vi "BIN_File.vi"(6 "Enum":enum16{"Read", "Write"}(ring), 8 "error in":errorcluster, 10 "Data":string, 11 "Path":path) -> (0 "error out":errorcluster, 2 "data out":string)   [LabVIEW 2024, in "Launcher_DTU.lvlib"]
uses:
  Launcher_DTU.lvlib
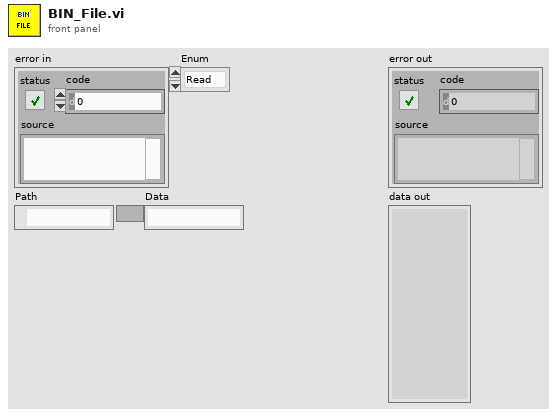
[diagram p1: front panel]
types:
  T1 = enum16{"open", "replace", "create", "open or create", "replace or create", "replace or create with confirmation"}
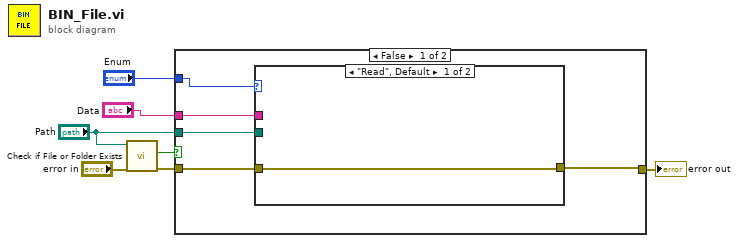
[diagram p0: block diagram]
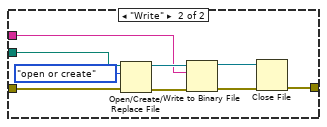
[diagram p2: hidden frame]
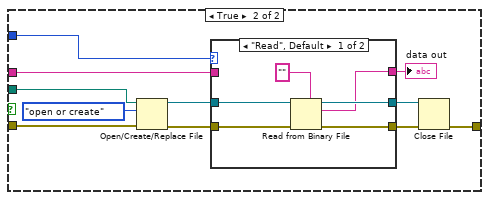
[diagram p3: hidden frame]
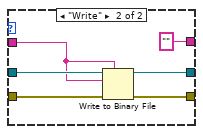
[diagram p4: hidden frame]
diagram:
  n1 = call <vilib>:"Check if File or Folder Exists.vi"("error in (no error)"="error in", "path"="Path") -> ("error out"=w6:errorcluster, "file or folder exists?"=w5:bool)  [unwired: 7 in, 1 out]
  n2 = case shown="False" w5 {
    tunnel: w6 -> [w11 w33]
    tunnel: "Path" -> [w10 w32]
    tunnel: [w8 w27] -> w3
    tunnel: "Data" -> [w9 w25]
    tunnel: "Enum" -> [w12 w24]
    frame False {
      n3 = case shown="\"Read\", Default" w12 {
        tunnel: w11 -> [w13 w22]
        tunnel: w10 -> [_ w21]
        tunnel: w9 -> [_ w17]
        tunnel: [w13 w14] -> w8
        frame "Read", Default {
        }
        frame "Write" {
          n4 = Open/Create/Replace File(file path (use dialog)=w21, error in=w22, operation (0:open)=T1."open or create") -> (refnum out=w18:refnum<file>, error out=w19:errorcluster)  [unwired: 3 in, 1 out]
          n5 = Write to Binary File(file (use dialog)=w18, data=w17, error in=w19) -> (refnum out=w16:refnum<file>, error out=w15:errorcluster)  [unwired: 3 in, 1 out]
          n6 = Close File(refnum=w16, error in=w15) -> (error out=w14:errorcluster)  [unwired: 1 out]
        }
      }
    }
    frame True {
      n7 = Open/Create/Replace File(file path (use dialog)=w32, error in=w33, operation (0:open)=T1."open or create") -> (refnum out=w28:refnum<file>, error out=w30:errorcluster)  [unwired: 3 in, 1 out]
      n8 = case shown="\"Read\", Default" w24 {
        tunnel: w30 -> [w39 w45]
        tunnel: [w38 w44] -> w29
        tunnel: w28 -> [w37 w43]
        tunnel: [w36 w42] -> w26
        tunnel: w25 -> [_ w41]
        tunnel: [w34 ""] -> w23
        frame "Read", Default {
          n9 = Read from Binary File(5:"" ("data type"), 8:w39, 11:w37) -> (0:w38:errorcluster, 2:w34:string, 3:w36:refnum<file>)  [unwired: 3 in, 1 out]
        }
        frame "Write" {
          n10 = Write to Binary File(file (use dialog)=w43, data=w41, error in=w45, 7:w41) -> (refnum out=w42:refnum<file>, error out=w44:errorcluster)  [unwired: 2 in, 1 out]
        }
      }
      "data out" <- w23
      n11 = Close File(refnum=w26, error in=w29) -> (error out=w27:errorcluster)  [unwired: 1 out]
    }
  }
  "error out" <- w3
